vi "TakeScaleCalibrationImage.vi"(8 "Error In":errorcluster, 9 "ExposureTime_us":u32, 10 "TLCamera reference in":refnum<k24>, 11 "MotorController in":refnum<class "MotorController.lvclass">) -> (0 "Error Out":errorcluster, 2 "TLCamera reference out":refnum<k24>, 3 "MotorController out":refnum<class "MotorController.lvclass">)   [LabVIEW 2019]
uses:
  C:/Users/jleeman/git_repos/CAxis_Machine/C-Axis LabView Controller/Library_X64/Thorlabs.TSI.TLCameraInterfaces.dll
  Library_X64/Thorlabs.TSI.TLCameraInterfaces.dll
  MotorController.lvclass
  TakeScaleCalibrationImage_states_enum_typedef.ctl
panel:
  out "mm/pixel":dbl
  in  "Real Distance (mm)":dbl
  out "Image":T1(plugin-control)
  in  "Calculate":bool
  in  "Next":bool
  # "Scale Calibration"
  # "1. Create two rectangular ROIs around the left and right most columns of visible holes in the grid. Hold ctrl to select the second area.\n2. Enter the actual distance in mm between the selected columns\n3. Click calculate\n4. Record the value"
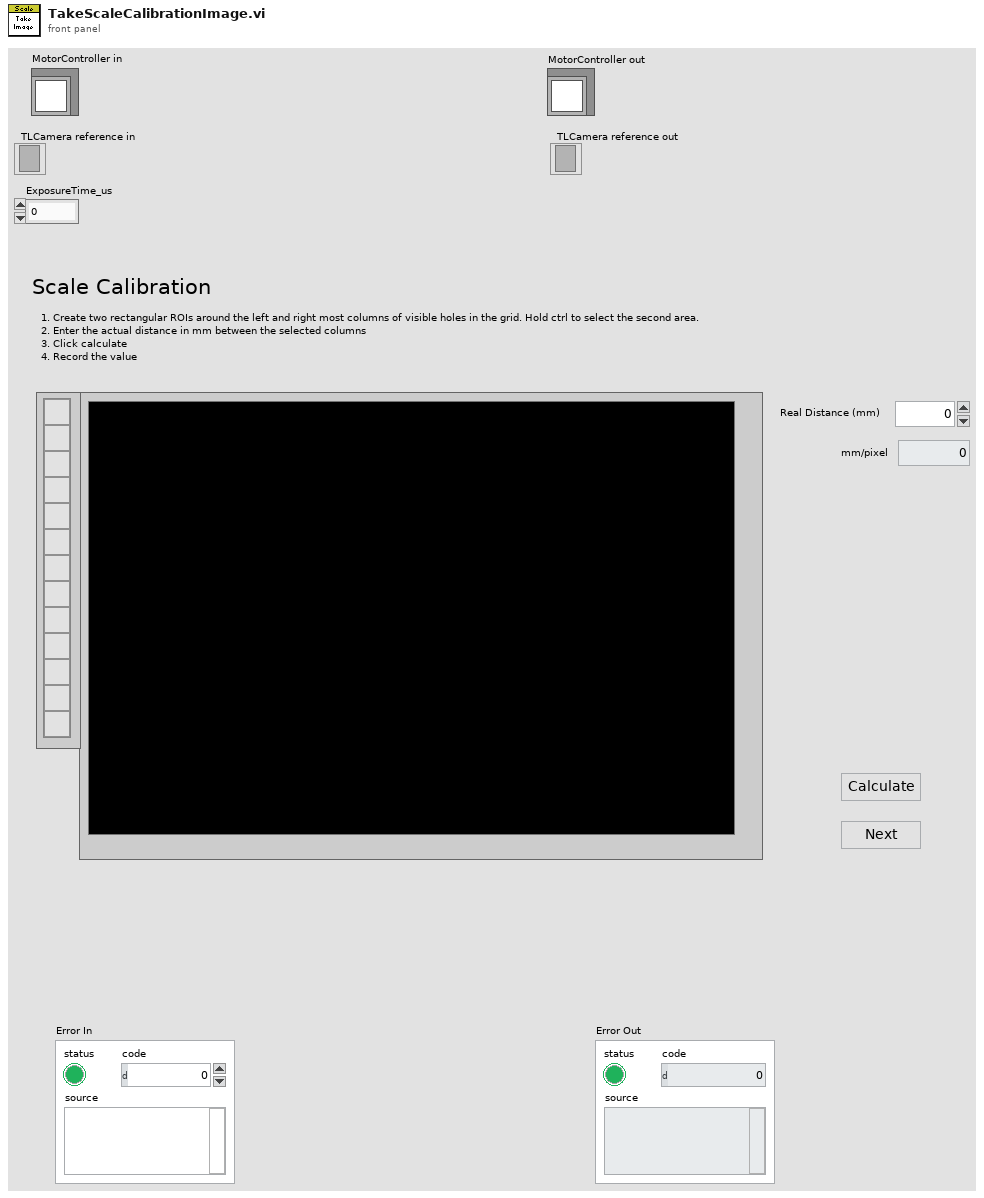
[diagram p1: front panel]
types:
  T1 = typedef "IMAQ Image.ctl" = refnum<image>
  T2 = typedef "Image Type" = u32
  T3 = typedef "TakeScaleCalibrationImage_states_enum_typedef.ctl" = enum16{"Calculate", "Initialize", "TakePhoto", "Wait", "Shutdown"}
  T4 = cluster{"Global Rectangle":i32[], "Contours":cluster{"Contour Type":u32, "ROI Type":u32, "Points":i32[]}[]}
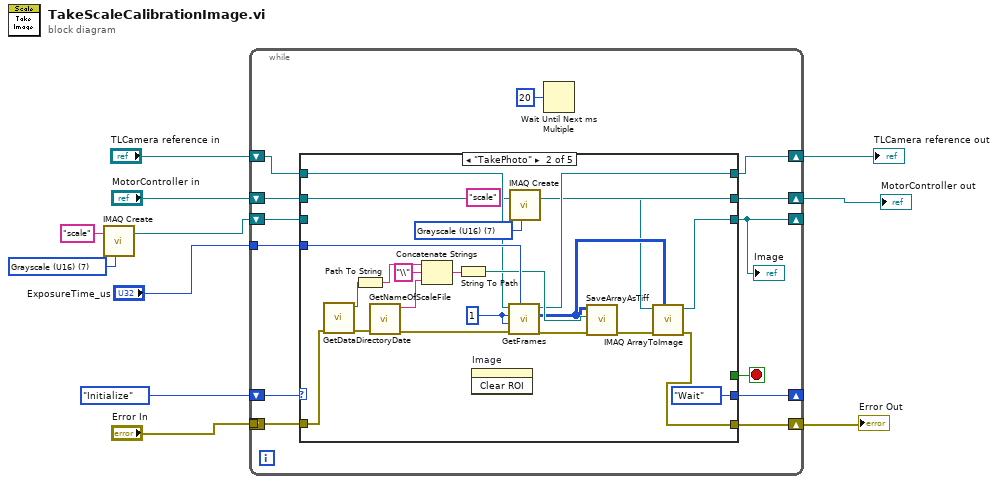
[diagram p0: block diagram]
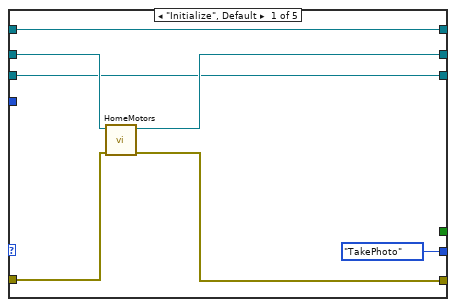
[diagram p2: hidden frame]
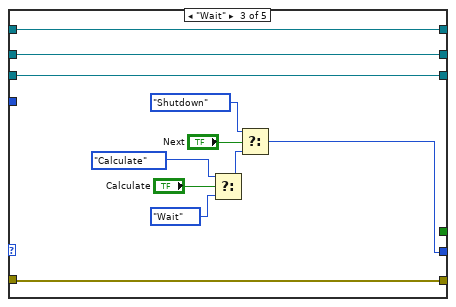
[diagram p3: hidden frame]
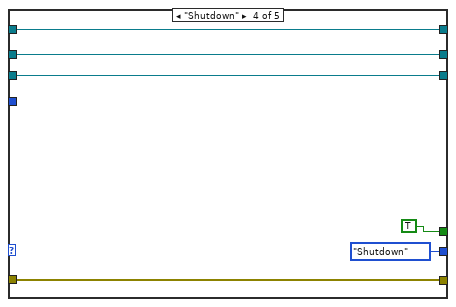
[diagram p4: hidden frame]
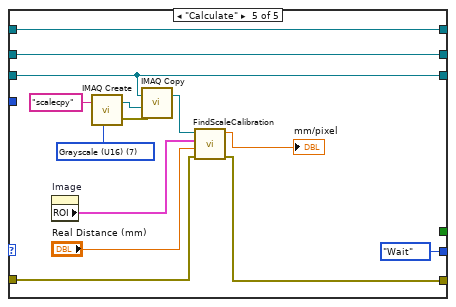
[diagram p5: hidden frame]
diagram:
  w2 = T2 7 items=["Grayscale (U8)", "Grayscale (I16)", "Grayscale (SGL)", "Complex (CSG)", "RGB (U32)", "HSL (U32)", "RGB (U64)", "Grayscale (U16)"] ("Image Type")
  n1 = call "IMAQ Create"("Image Name"="scale", "Image Type"=w2) -> ("New Image"=w1:T1)  [unwired: 3 in, 1 out]
  n2 = while {
    shift-right: [w23] -> _
    shift-left: TakeScaleCalibrationImage_states_enum_typedef."Initialize" -> [w24]
    shift-right: [w19] -> w4
    shift-left: "MotorController in" -> [w21]
    shift-right: [w16] -> w8
    shift-left: "TLCamera reference in" -> [w17]
    tunnel: "Error In" -> [w20]
    shift-right: [w18] -> w6
    shift-left: _ -> [_]
    tunnel: "ExposureTime_us" -> [w15]
    shift-right: [w12] -> _
    shift-left: w1 -> [w13]
    stop <- w14 stop-if-true
    n3 = case shown="\"TakePhoto\"" w24 {
      tunnel: [TakeScaleCalibrationImage_states_enum_typedef."TakePhoto" TakeScaleCalibrationImage_states_enum_typedef."Wait" w63 TakeScaleCalibrationImage_states_enum_typedef."Shutdown" TakeScaleCalibrationImage_states_enum_typedef."Wait"] -> w23
      tunnel: w21 -> [w30 w39 w61 w70 w80]
      tunnel: w20 -> [w29 w54 w62 w69 w81]
      tunnel: [w27 w39 w61 w70 w80] -> w19
      tunnel: [w26 w35 w62 w69 w82] -> w18
      tunnel: w17 -> [w28 w40 w60 w71 w79]
      tunnel: [w28 w41 w60 w71 w79] -> w16
      tunnel: w15 -> [_ w45 _ _ _]
      tunnel: [_ _ _ TRUE _] -> w14
      tunnel: w13 -> [w25 _ w59 w66 w76]
      tunnel: [w25 w37 w59 w66 w76] -> w12
      frame "Initialize", Default {
        n4 = call "HomeMotors.vi"("error in (no error)"=w29, "MotorController in"=w30) -> ("error out"=w26:errorcluster, "MotorController out"=w27:refnum<class "MotorController.lvclass">)  [unwired: 8 in]
      }
      frame "TakePhoto" {
        w33 = T2 7 items=["Grayscale (U8)", "Grayscale (I16)", "Grayscale (SGL)", "Complex (CSG)", "RGB (U32)", "HSL (U32)", "RGB (U64)", "Grayscale (U16)"] ("Image Type")
        w46 = u32 1 ("Gain")
        n5 = call "GetDataDirectoryDate.vi"("Error In"=w54) -> ("Error Out"=w53:errorcluster, "path"=w51:path)  [unwired: 9 in]
        n6 = Path To String(path=w51) -> (string=w50:string)
        n7 = call "GetNameOfScaleFile.vi"("Error In"=w53) -> ("Error Out"=w52:errorcluster, "Scale Filename"=w48:string)  [unwired: 9 in]
        n8 = Concatenate Strings(w50, "\\" ("string"), w48) -> (w47:string)
        n9 = String To Path(string=w47) -> (path=w44:path)
        n10 = invoke on="Image" class="ImageControl" method="Clear ROI"() -> ()  [unwired: 3 in, 3 out]
        n11 = call "GetFrames.vi"("ExposureTime_us"=w45, "Error In"=w52, "FramesPerTrigger"=w46, "Gain"=w46, "TLCamera reference in"=w40) -> ("Error Out"=w43:errorcluster, "Array"=w38:u16[][], "TLCamera reference out"=w41:refnum<k24>)  [unwired: 4 in]
        n12 = call "IMAQ Create"("Image Name"="scale", "Image Type"=w33) -> ("New Image"=w32:T1)  [unwired: 3 in, 1 out]
        n13 = call "SaveArrayAsTiff.vi"("Error In"=w43, "File Path"=w44, "Array"=w38) -> ("Error Out"=w36:errorcluster)  [unwired: 7 in, 1 out]
        n14 = call "IMAQ ArrayToImage"("Image Pixels (U16)"=w38, "error in (no error)"=w36, "Image"=w32) -> ("error out"=w35:errorcluster, "Image Out"=w37:T1)  [unwired: 7 in]
      }
      frame "Wait" {
        n15 = Select(t=TakeScaleCalibrationImage_states_enum_typedef."Calculate", s="Calculate", f=TakeScaleCalibrationImage_states_enum_typedef."Wait") -> (s? t:f=w55:T3)
        n16 = Select(t=TakeScaleCalibrationImage_states_enum_typedef."Shutdown", s="Next", f=w55) -> (s? t:f=w63:T3)
      }
      frame "Shutdown" {
      }
      frame "Calculate" {
        w73 = T2 7 items=["Grayscale (U8)", "Grayscale (I16)", "Grayscale (SGL)", "Complex (CSG)", "RGB (U32)", "HSL (U32)", "RGB (U64)", "Grayscale (U16)"] ("Image Type")
        n17 = property on="Image" class="ImageControl"() -> ("ROI"=w85:T4)  [unwired: 2 in, 2 out]
        n18 = call "IMAQ Create"("Image Name"="scalecpy", "Image Type"=w73) -> ("New Image"=w75:T1, "error out"=w74:errorcluster)  [unwired: 3 in]
        n19 = call "IMAQ Copy"("error in (no error)"=w74, "Image Dst"=w75, "Image Src"=w76) -> ("Image Dst Out"=w77:T1)  [unwired: 3 in, 1 out]
        n20 = call "FindScaleCalibration.vi"("Error In"=w81, "mm"="Real Distance (mm)", "ROI Descriptor"=w85, "Image Src"=w77) -> ("Error Out"=w82:errorcluster, "mm/pix"=→"mm/pixel":sgl)  [unwired: 6 in]
      }
    }
    "Image" <- w12
    n21 = Wait Until Next ms Multiple(millisecond multiple=u32 20) -> ()  [unwired: 1 out]
  }
  "TLCamera reference out" <- w8
  "Error Out" <- w6
  "MotorController out" <- w4
